vi "SimpleSerialTest_with_regex.vi"() -> ()   [LabVIEW 2013]
uses:
  Data/TypeDefs/Notifiers.ctl
  Data/TypeDefs/UTM Location.ctl
  Data/TypeDefs/Sail Set Suggestions.ctl
  Data/TypeDefs/Rudder Set Suggestions.ctl
  Data/TypeDefs/OverrideInformation.ctl
  Data/TypeDefs/OverrideMode.ctl
  Data/TypeDefs/MotorSetup.ctl
  Data/TypeDefs/DynamixelSetupInfo.ctl
  Data/TypeDefs/AirmarStatus.ctl
  Data/TypeDefs/HardwareOnline.ctl
  Data/TypeDefs/DynamixelCycleTracker.ctl
  Data/TypeDefs/RC Input Values.ctl
  Classes/Waypoint/Waypoint.lvclass
  <vilib>/regexp/Match Regular Expression.xnode
  <vilib>/Instr/_visa.llb/VISA Configure Serial Port (Instr).vi
  Data/TypeDefs/GPS-Compass Queue Cluster.ctl
  Data/TypeDefs/WindData Queue Cluster.ctl
panel:
  out "Loop Frequency":dbl(graph)
  out "Loop Frequency (Hz)":dbl
  in  "Cycles per buffer flush":i32=1000
  out "Sentence":string
  in  "stop":bool
  out "While counter":i32
  in  "NotifierReff":T1
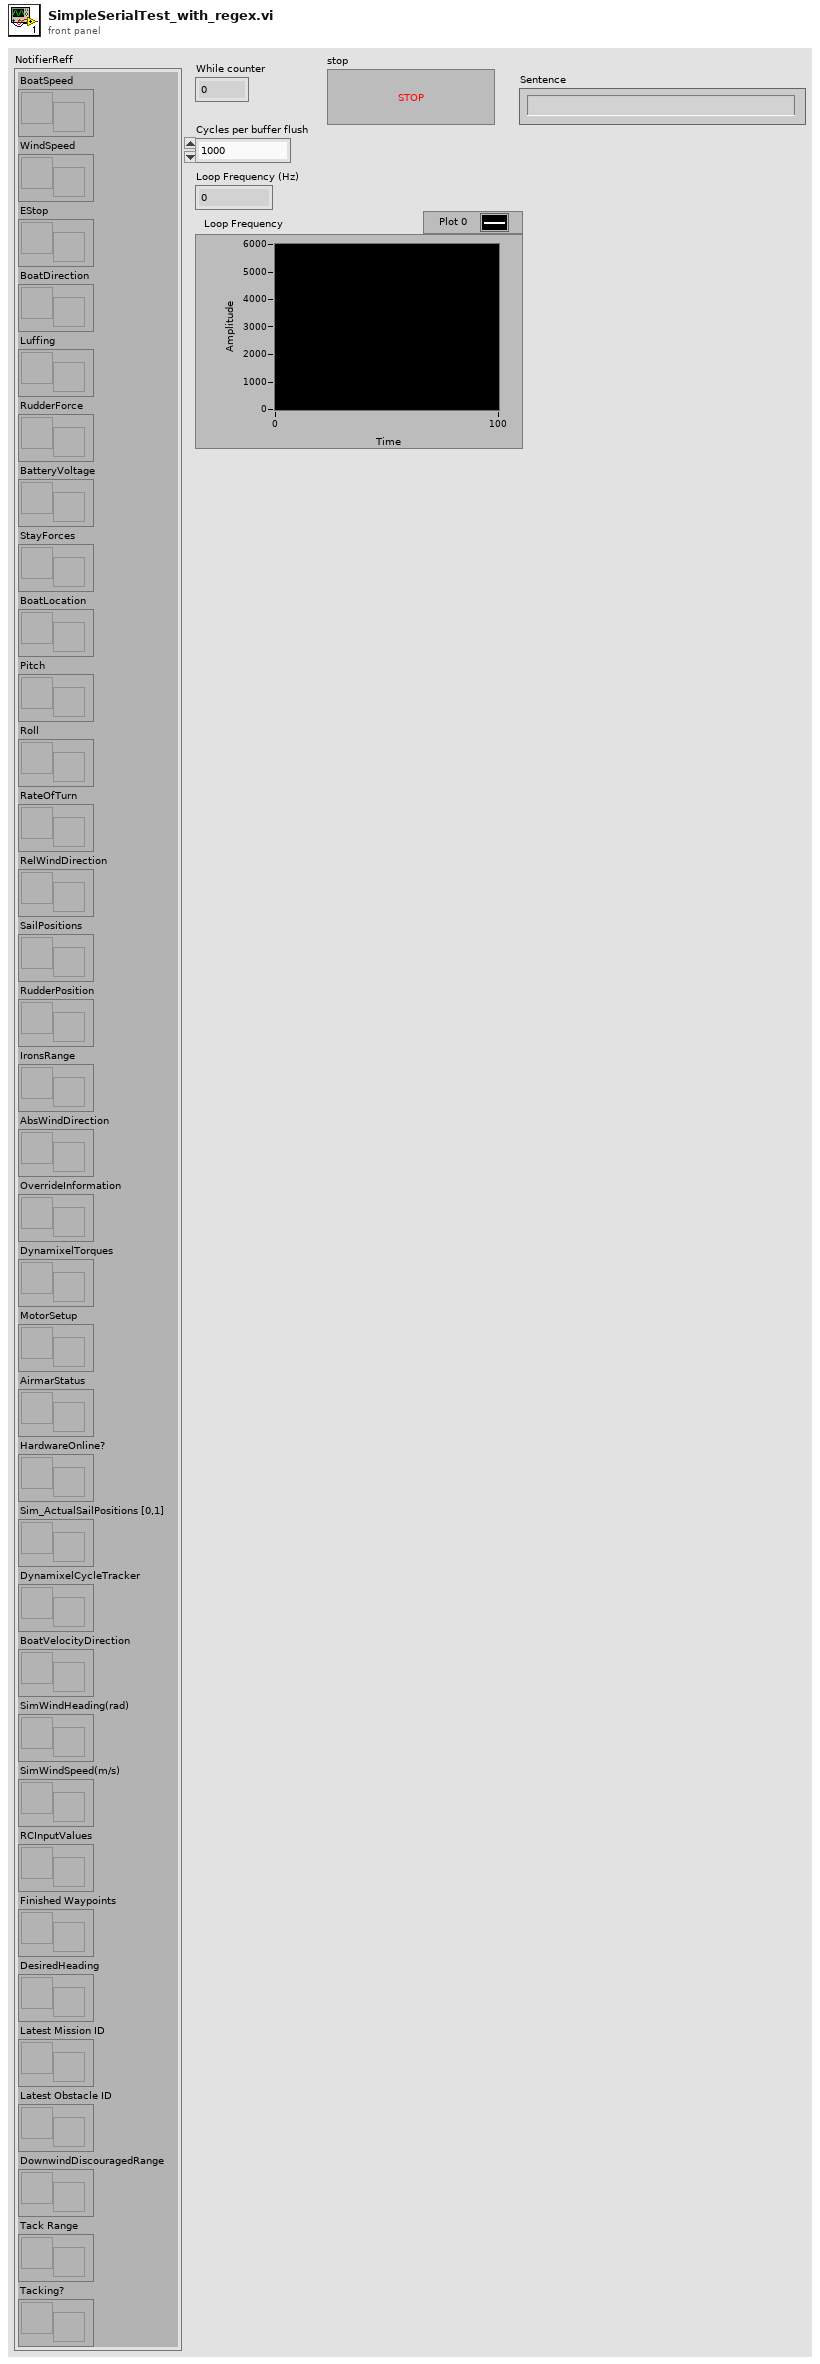
[diagram p1: front panel]
types:
  T1 = typedef "Notifiers.ctl" = cluster{"BoatSpeed":refnum<notifier>, "WindSpeed":refnum<notifier>, "EStop":refnum<notifier>, "BoatDirection":refnum<notifier>, "Luffing":refnum<notifier>, "RudderForce":refnum<notifier>, "BatteryVoltage":refnum<notifier>, "StayForces":refnum<notifier>, "BoatLocation":refnum<notifier>, "Pitch":refnum<notifier>, "Roll":refnum<notifier>, "RateOfTurn":refnum<notifier>, "RelWindDirection":refnum<notifier>, "SailPositions":refnum<notifier>, "RudderPosition":refnum<notifier>, "IronsRange":refnum<notifier>, "AbsWindDirection":refnum<notifier>, "OverrideInformation":refnum<notifier>, "DynamixelTorques":refnum<notifier>, "MotorSetup":refnum<notifier>, "AirmarStatus":refnum<notifier>, "HardwareOnline?":refnum<notifier>, "Sim_ActualSailPositions [0,1]":refnum<notifier>, "DynamixelCycleTracker":refnum<notifier>, "BoatVelocityDirection":refnum<notifier>, "SimWindHeading(rad)":refnum<notifier>, "SimWindSpeed(m/s)":refnum<notifier>, "RCInputValues":refnum<notifier>, "Finished Waypoints":refnum<notifier>, "DesiredHeading":refnum<notifier>, "Latest Mission ID":refnum<notifier>, "Latest Obstacle ID":refnum<notifier>, "DownwindDiscouragedRange":refnum<notifier>, "Tack Range":refnum<notifier>, "Tacking?":refnum<notifier>}
  T2 = typedef "WindData Queue Cluster.ctl" = cluster{"RelWindDirection Queue":refnum<queue>, "WindSpeed Queue":refnum<queue>, "AbsWindDirection Queue":refnum<queue>}
  T3 = typedef "GPS-Compass Queue Cluster.ctl" = cluster{"BoatLocation Queue":refnum<queue>, "BoatDirection Queue":refnum<queue>, "BoatSpeed Queue":refnum<queue>, "RateOfTurn Queue":refnum<queue>, "Pitch Queue":refnum<queue>, "Roll Queue":refnum<queue>, "BoatVelocityDirection Queue ":refnum<queue>}
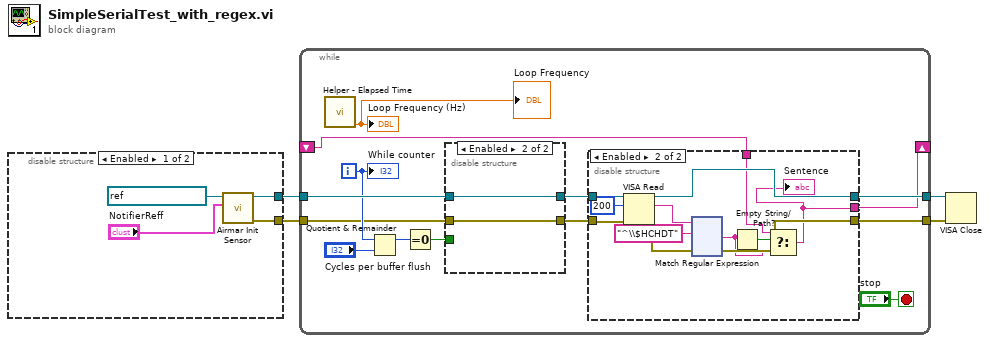
[diagram p0: block diagram]
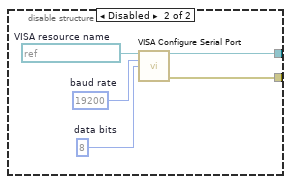
[diagram p2: hidden frame]
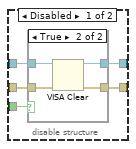
[diagram p3: hidden frame]
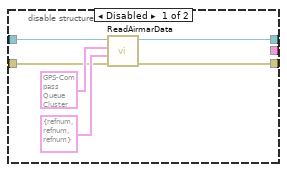
[diagram p5: hidden frame]
diagram:
  n1 = disable-structure shown="Enabled" {
    disable-tunnel: [w6 w10] -> w4
    disable-tunnel: [w5 w9] -> w2
    frame Enabled {
      n2 = call "Airmar Init Sensor.vi"("NotifierReff"="NotifierReff", "VISA Refnum in"=refnum<visa-resource-name> "ASRL2::INSTR") -> ("error out"=w5:errorcluster, "VISA Refnum out"=w6:refnum<visa-resource-name>)  [unwired: 7 in, 1 out]
    }
    frame Disabled {
      w13 = u16 8  # data bits
      w11 = u32 19200  # baud rate
      w12 = refnum<visa-resource-name> "ASRL1::INSTR"  # VISA resource name
      n3 = call-poly "VISA Configure Serial Port"("VISA resource name"=w12, "baud rate (9600)"=w11, "data bits (8)"=w13) -> ("VISA resource name out"=w10:refnum<visa-resource-name>, "error out"=w9:errorcluster)  [unwired: 11 in]
    }
  }
  n4 = while {
    tunnel: w4 -> [w26]
    tunnel: [w20] -> w3
    tunnel: w2 -> [w18]
    tunnel: [w16] -> w1
    shift-right: [w15] -> _
    shift-left: _ -> [w14]
    i -> [w25]
    stop <- "stop" stop-if-true
    n5 = call "Helper - Elapsed Time.vi"() -> ("Frequency (Hz)"=→"Loop Frequency (Hz)" →"Loop Frequency":dbl)  [unwired: 10 in, 1 out]
    n6 = Quotient & Remainder(x=w25, y="Cycles per buffer flush") -> (x-y*floor(x/y)=w24:i32)  [unwired: 1 out]
    n7 = Equal To 0?(x=w24) -> (x = 0?=w23:bool)
    n8 = disable-structure shown="Enabled" {
      disable-tunnel: [w32 w40] -> w19
      disable-tunnel: w26 -> [w31 w40]
      disable-tunnel: w23 -> [w30 _]
      disable-tunnel: w18 -> [w29 w39]
      disable-tunnel: [w28 w39] -> w17
      frame Disabled {
        n9 = case shown="True" w30 {
          tunnel: [w34 w38] -> w32
          tunnel: w31 -> [w34 w37]
          tunnel: w29 -> [w33 w36]
          tunnel: [w33 w35] -> w28
          frame False {
          }
          frame True {
            n10 = VISA Clear(VISA resource name=w37, error in (no error)=w36) -> (VISA resource name out=w38:refnum<visa-resource-name>, error out=w35:errorcluster)
          }
        }
      }
      frame Enabled {
      }
    }
    n11 = disable-structure shown="Enabled" {
      disable-tunnel: w19 -> [w46 w58]
      disable-tunnel: [w43 w53] -> w20
      disable-tunnel: w17 -> [w42 w57]
      disable-tunnel: [w41 w52] -> w16
      disable-tunnel: [_ w48] -> w15
      disable-tunnel: w14 -> [_ w47]
      frame Disabled {
        n12 = call "ReadAirmarData.vi"("Error in"=w42, "Airmar Wind Queue Cluster"=T2 {"RelWindDirection Queue"=refnum, "WindSpeed Queue"=refnum, "AbsWindDirection Queue"=refnum}, "AirmarGPS-Compass Queue Cluster"=T3 {"BoatLocation Queue"=refnum, "BoatDirection Queue"=refnum, "BoatSpeed Queue"=refnum, "RateOfTurn Queue"=refnum, "Pitch Queue"=refnum, "Roll Queue"=refnum, "BoatVelocityDirection Queue "=refnum}, "VISA UART port"=w46) -> ("Error out"=w41:errorcluster, "VISA UART port Out"=w43:refnum<visa-resource-name>)  [unwired: 5 in, 1 out]
      }
      frame Enabled {
        n13 = VISA Read(VISA resource name=w58, byte count=u32 200, error in (no error)=w57) -> (VISA resource name out=w53:refnum<visa-resource-name>, read buffer=w55:string, error out=w51:errorcluster)  [unwired: 1 out]
        n14 = xnode "Match Regular Expression"("input string"=w55, "regular expression"="^\\$HCHDT", "error in"=w51) -> ("after match"=w49:string, "error out"=w52:errorcluster)  [unwired: 3 in, 3 out]
        n15 = Empty String/Path?(string/path=w49) -> (empty?=w50:bool)
        n16 = Select(t=w47, s=w50, f=w49) -> (s? t:f=w48:string)
        "Sentence" <- w48
      }
    }
    "While counter" <- w25
  }
  n17 = VISA Close(VISA resource name=w3, error in (no error)=w1) -> ()  [unwired: 1 out]
